vi "PID.vi"(1 "Present Value":dbl=15.0 format="%.2f", 3 "Setpoint":dbl=15.0 format="%.2f") -> (0 "Dem Output":dbl format="%.2f")   [LabVIEW 2011]
uses:
  <vilib>/Analysis/NI_AALPro.lvlib
panel:
  in  "O/P deadband":dbl=1.0 format="%.2f"
  in  "Kp Deadband":dbl format="%.2f"
  in  "Derivative History":i32=20
  out "deadbanded error":dbl format="%.2f"
  in  "P":bool=TRUE
  in  "D":bool=TRUE
  in  "I":bool=TRUE
  out "Waveform Chart":T1(graph)
  in  "Manual Demand":dbl min=0.0 max=100.0 format="%.2f"
  in  "Manual Override":bool
  out "Control Sum":dbl format="%.2f"
  out "Derivative Term":dbl format="%.2f"
  out "Integral Term":dbl format="%.2f"
  out "error differential":dbl format="%.5f"
  out "error integral":dbl format="%.2f"
  out "Proportional Term":dbl format="%.2f"
  in  "Kd":dbl=50.0 format="%.2f"
  in  "Ki":dbl=0.03 format="%.3f"
  in  "Kp":dbl=5.0 format="%.2f"
  out "error":dbl format="%.2f"
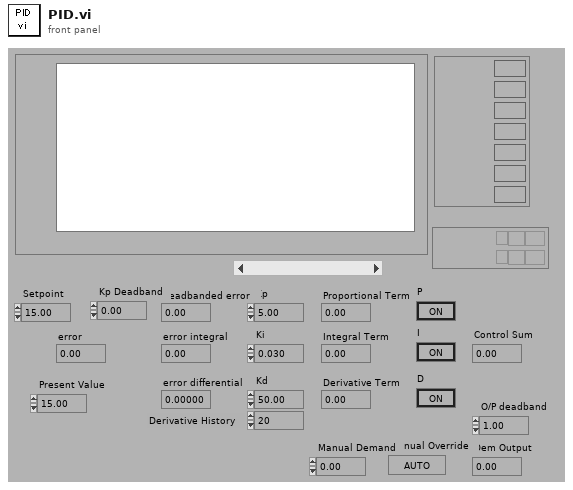
[diagram p1: front panel]
types:
  T1 = cluster{"Setpoint":dbl, "Present Value":dbl, "Proportional Term":dbl, "Integral Term":dbl, "Derivative Term":dbl, "Control Sum":dbl, "Dem Output":dbl}
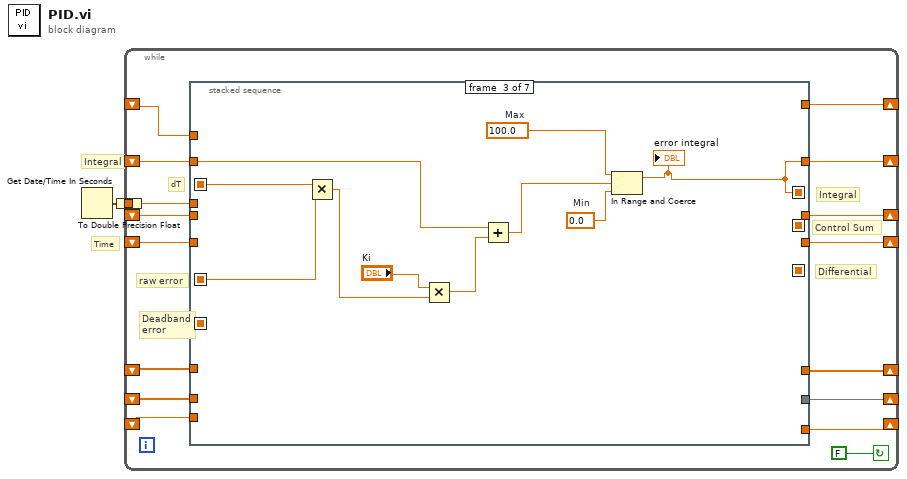
[diagram p0: block diagram]
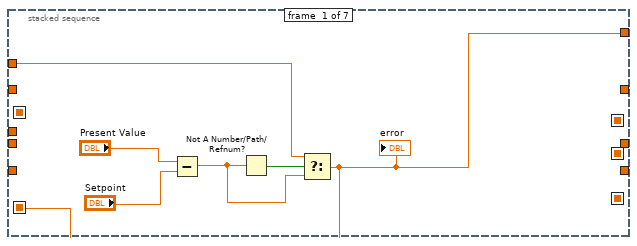
[diagram p2: hidden frame]
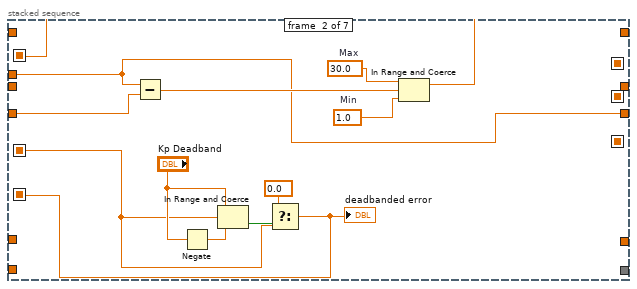
[diagram p3: hidden frame]
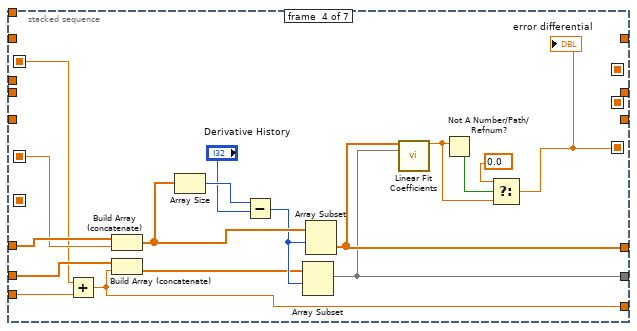
[diagram p4: hidden frame]
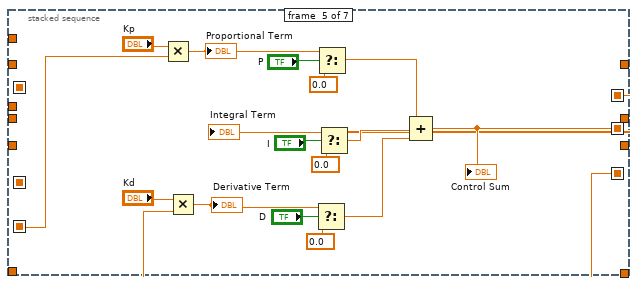
[diagram p5: hidden frame]
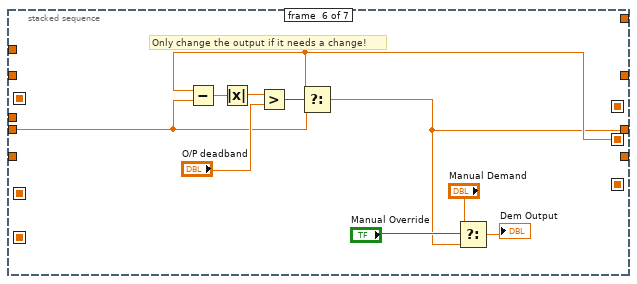
[diagram p6: hidden frame]
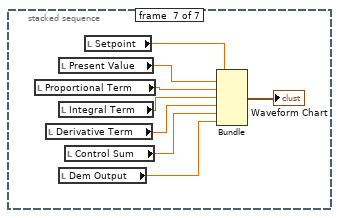
[diagram p7: hidden frame]
diagram:
  # "Integral"
  # "Time"
  n1 = Get Date/Time In Seconds() -> (seconds since 1Jan1904=w1:timestamp)
  n2 = To Double Precision Float(number=w1) -> (double precision float=w2:dbl)
  n3 = while {
    shift-left: _ -> [w5]
    shift-right: [w4] -> _
    shift-left: _ -> [w7]
    shift-right: [w6] -> _
    shift-left: _ -> [w9]
    shift-right: [w8] -> _
    tunnel: w2 -> [w14]
    shift-left: _ -> [w11]
    shift-right: [w10] -> _
    shift-left: _ -> [w13]
    shift-right: [w12] -> _
    shift-left: _ -> [w15]
    shift-right: [w16] -> _
    shift-left: _ -> [w18]
    shift-right: [w17] -> _
    stop <- FALSE continue-if-true
    # "Control Sum"
    # "raw error"
    # "Differential"
    # "Integral"
    # "Deadband\nerror"
    # "dT"
    n4 = stacked-sequence {
      seq-local: [_ w25 _ _ _ _ _] -> [_ _ w46 w49 _ _ _]
      seq-local: [_ w34 _ _ _ _ _] -> [_ _ _ _ w66 _ _]
      seq-local: [_ _ _ w54 _ _ _] -> [_ _ _ _ w65 _ _]
      seq-local: [_ _ w41 _ _ _ _] -> [_ _ _ _ w64 _ _]
      seq-local: [w19 _ _ _ _ _ _] -> [_ w26 w43 w55 _ _ _]
      seq-local: [_ _ _ _ w69 _ _] -> [_ _ _ _ _ w84 _]
      tunnel: w18 -> [_ w31 _ _ _ _ _]
      tunnel: [_ w29 _ _ _ _ _] -> w17
      tunnel: [_ _ w41 _ _ _ _] -> w16
      tunnel: w15 -> [_ _ w38 _ _ _ _]
      tunnel: w14 -> [_ w29 _ _ _ _ _]
      tunnel: w13 -> [_ _ _ w63 _ _ _]
      tunnel: [_ _ _ w56 _ _ _] -> w12
      tunnel: w11 -> [_ _ _ w62 _ _ _]
      tunnel: [_ _ _ w53 _ _ _] -> w10
      tunnel: w9 -> [_ _ _ _ _ w82 _]
      tunnel: [_ _ _ _ _ w81 _] -> w8
      tunnel: w7 -> [_ _ _ w48 _ _ _]
      tunnel: [_ _ _ w47 _ _ _] -> w6
      tunnel: w5 -> [w21 _ _ _ _ _ _]
      tunnel: [w19 _ _ _ _ _ _] -> w4
      frame #0 {
        n5 = Subtract(x="Present Value", y="Setpoint") -> (x-y=w20:dbl)
        n6 = Not A Number/Path/Refnum?(number/path/refnum=w20) -> (NaN/Path/Refnum?=w22:bool)
        n7 = Select(t=w21, s=w22, f=w20) -> (s? t:f=w19:dbl)
        "error" <- w19
      }
      frame #1 {
        w32 = 1.0  # Min
        w33 = 30.0  # Max
        n8 = Subtract(x=w29, y=w31) -> (x-y=w30:dbl)
        n9 = Negate(x="Kp Deadband") -> (-x=w28:dbl)
        n10 = In Range and Coerce(upper limit="Kp Deadband", x=w26, lower limit=w28) -> (In Range?=w35:bool)  [unwired: 1 out]
        n11 = Select(t=0.0, s=w35, f=w26) -> (s? t:f=w34:dbl)
        "deadbanded error" <- w34
        n12 = In Range and Coerce(upper limit=w33, x=w30, lower limit=w32) -> (coerced(x)=w25:dbl)  [unwired: 1 out]
      }
      frame #2 {
        w45 = 0.0  # Min
        w40 = 100.0  # Max
        n13 = Multiply(x=w46, y=w43) -> (x*y=w39:dbl)
        n14 = Multiply(x="Ki", y=w39) -> (x*y=w42:dbl)
        n15 = Add(x=w38, y=w42) -> (x+y=w44:dbl)
        n16 = In Range and Coerce(upper limit=w40, x=w44, lower limit=w45) -> (coerced(x)=w41:dbl)  [unwired: 1 out]
        "error integral" <- w41
      }
      frame #3 {
        n17 = Add(x=w49, y=w48) -> (x+y=w47:dbl)
        n18 = Build Array (concatenate)(w63, w55) -> (w59:dbl[])
        n19 = Build Array (concatenate)(w62, w47) -> (w57:dbl[])
        n20 = Array Size(array=w59) -> (size(s)=w61:i32)
        n21 = Subtract(x=w61, y="Derivative History") -> (x-y=w58:i32)
        n22 = Array Subset(array=w57, index=w58) -> (w53:dbl[])  [unwired: 1 in]
        n23 = Array Subset(array=w59, index=w58) -> (w56:dbl[])  [unwired: 1 in]
        n24 = call <vilib>:"Linear Fit Coefficients.vi"("Y"=w56, "X"=w53) -> ("slope"=w50:dbl)  [unwired: 3 in, 10 out]
        n25 = Not A Number/Path/Refnum?(number/path/refnum=w50) -> (NaN/Path/Refnum?=w52:bool)
        n26 = Select(t=0.0 ("f"), s=w52, f=w50) -> (s? t:f=w54:dbl)
        "error differential" <- w54
      }
      frame #4 {
        n27 = Multiply(x="Kp", y=w66) -> (x*y=w78:dbl)
        "Proportional Term" <- w78
        n28 = Multiply(x="Kd", y=w65) -> (x*y=w70:dbl)
        "Derivative Term" <- w70
        n29 = Select(t=w70, s="D", f=0.0) -> (s? t:f=w72:dbl)
        n30 = Select(t=w78, s="P", f=0.0) -> (s? t:f=w79:dbl)
        n31 = Select(t=w64, s="I", f=0.0) -> (s? t:f=w71:dbl)
        n32 = Compound Arithmetic op=ADD(w79, w71, w72) -> (w69:dbl)
        "Control Sum" <- w69
        "Integral Term" <- w64
      }
      frame #5 {
        # "Only change the output if it needs a change!"
        n33 = Subtract(x=w84, y=w82) -> (x-y=w87:dbl)
        n34 = Absolute Value(x=w87) -> (abs(x)=w86:dbl)
        n35 = Greater?(x=w86, y="O/P deadband") -> (0:w85:bool)
        n36 = Select(t=w84, s=w85, f=w82) -> (s? t:f=w81:dbl)
        n37 = Select(t="Manual Demand", s="Manual Override", f=w81) -> (s? t:f=→"Dem Output":dbl)
      }
      frame #6 {
        n38 = local read "Proportional Term"() -> (w94:dbl)
        n39 = local read "Derivative Term"() -> (w96:dbl)
        n40 = local read "Present Value"() -> (w93:dbl)
        n41 = local read "Integral Term"() -> (w95:dbl)
        n42 = local read "Dem Output"() -> (w98:dbl)
        n43 = local read "Control Sum"() -> (w97:dbl)
        n44 = local read "Setpoint"() -> (w92:dbl)
        n45 = Bundle("Setpoint"=w92, "Present Value"=w93, "Proportional Term"=w94, "Integral Term"=w95, "Derivative Term"=w96, "Control Sum"=w97, "Dem Output"=w98) -> (→"Waveform Chart":T1)  [unwired: 1 out]
      }
    }
  }
